vi "Get ROI Array.vi"(0 "Image Ref":T1, 11 "Error In":errorcluster) -> (4 "Image Out":u16[][](array[numeric]), 15 "Error Out":errorcluster)   [LabVIEW 2020]
uses:
  <vilib>/vision/Image Controls.llb/IMAQ Image.ctl
  Display Module Custom Controls/ROI Descriptor.ctl
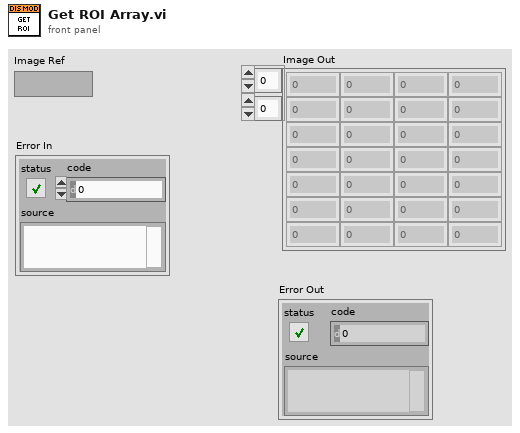
[diagram p1: front panel]
types:
  T1 = typedef "IMAQ Image.ctl" = refnum<image>
  T2 = typedef "ROI Descriptor.ctl" = cluster{"Global Rectangle":i32[], "Contours":cluster{"Contour Type":u32, "ROI Type":u32, "Points":i32[]}[]}
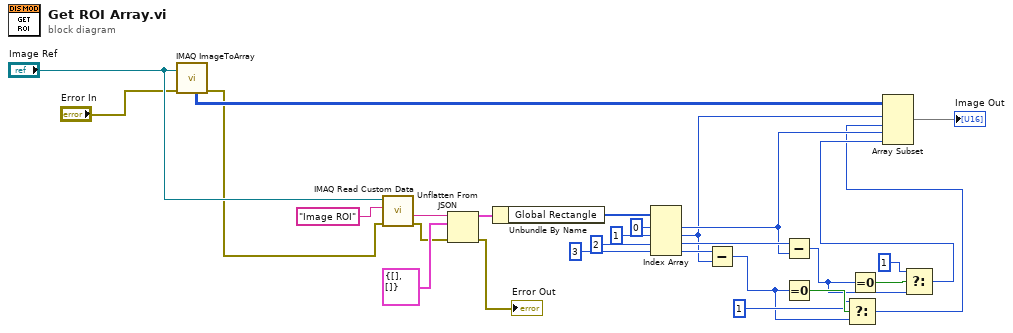
[diagram p0: block diagram]
diagram:
  n1 = call "IMAQ ImageToArray"("error in (no error)"="Error In", "Image"="Image Ref") -> ("Image Pixels (U16)"=w19:u16[][], "error out"=w3:errorcluster)  [unwired: 2 in, 3 out]
  n2 = call "IMAQ Read Custom Data"("error in (no error)"=w3, "Key"="Image ROI", "Image"="Image Ref") -> ("error out"=w2:errorcluster, "Custom Data Out"=w27:string)  [unwired: 6 in, 1 out]
  n3 = Unflatten From JSON(JSON string=w27, type and defaults=T2 {"Global Rectangle"=[], "Contours"=[]} ("Image ROI Descriptor"), error in (no error)=w2) -> (value=w25:T2, error out=→"Error Out":errorcluster)  [unwired: 4 in]
  n4 = Unbundle By Name(w25) -> ("Global Rectangle"=w24:i32[])
  n5 = Index Array(array=w24, index #1=0 ("index"), index #2=1 ("index"), index #3=2 ("index"), index #4=3 ("index")) -> (element #1=w16:i32, element #2=w15:i32, element #3=w18:i32, element #4=w17:i32)
  n6 = Subtract(x=w17, y=w15) -> (x-y=w10:i32)
  n7 = Subtract(x=w18, y=w16) -> (x-y=w9:i32)
  n8 = Equal To 0?(x=w10) -> (x = 0?=w14:bool)
  n9 = Select(t=1 ("index"), s=w14, f=w10) -> (s? t:f=w7:i32)
  n10 = Equal To 0?(x=w9) -> (x = 0?=w13:bool)
  n11 = Select(t=1 ("index"), s=w13, f=w9) -> (s? t:f=w8:i32)
  n12 = Array Subset(array=w19, index (row)=w15, length (row)=w7, index (col)=w16, length (col)=w8) -> (→"Image Out":u16[][])
